vi "number1-state machine.vi"() -> ()   [LabVIEW 2014]
uses:
  number1_global.vi
panel:
  out "Numeric":i32
  out "index of element":i32
  out "Logined":bool
  in  "stop":bool
  out "array":bool[](array[boolean])
  in  "Button":T1
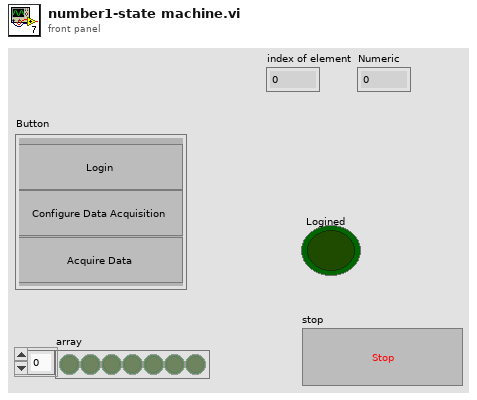
[diagram p1: front panel]
types:
  T1 = cluster{"OK Button":bool, "OK Button 2":bool, "OK Button 3":bool}
  T2 = enum32{"Invalid", "Standard", "Closed", "Hidden", "Minimized", "Maximized"}
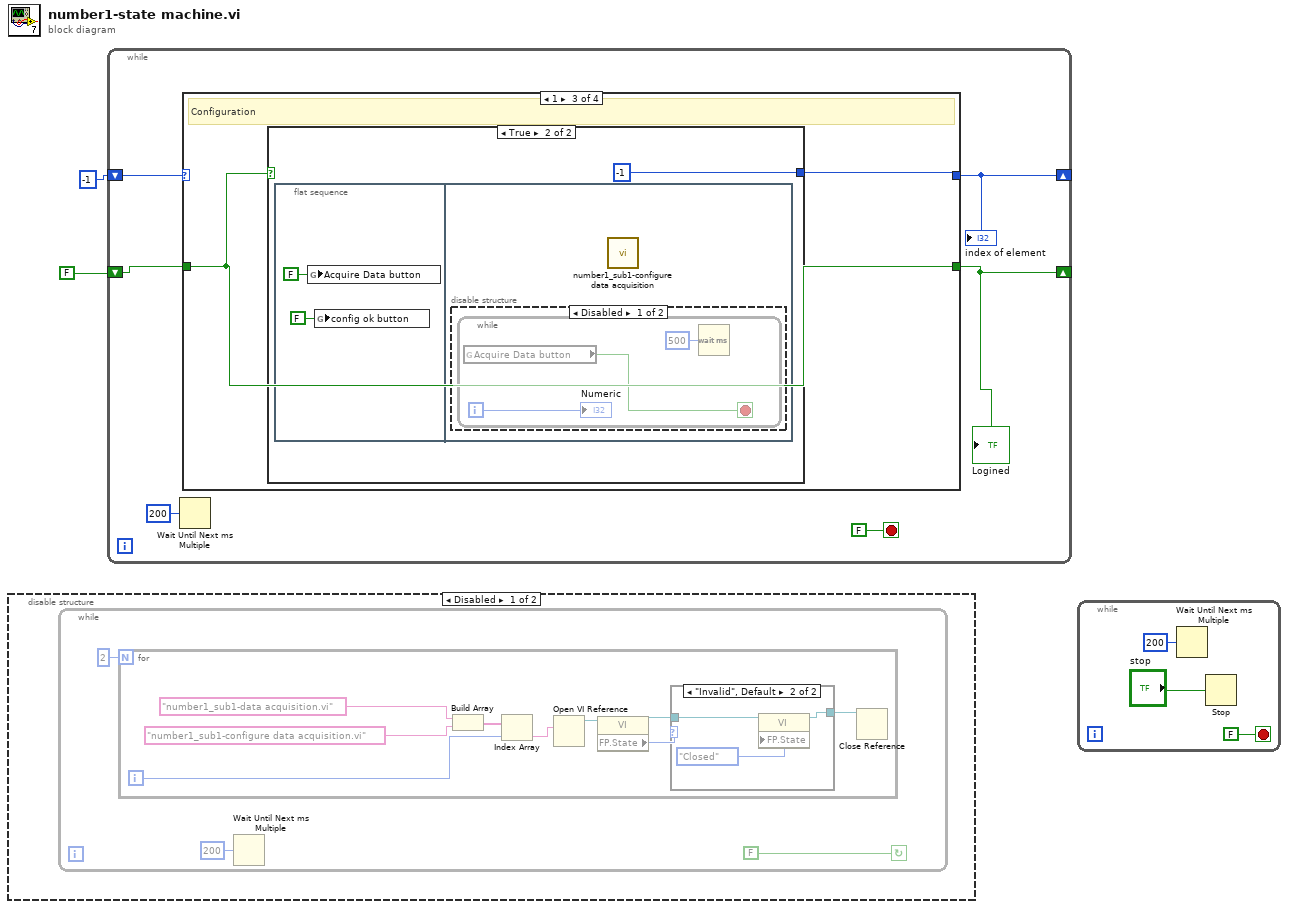
[diagram p0: block diagram]
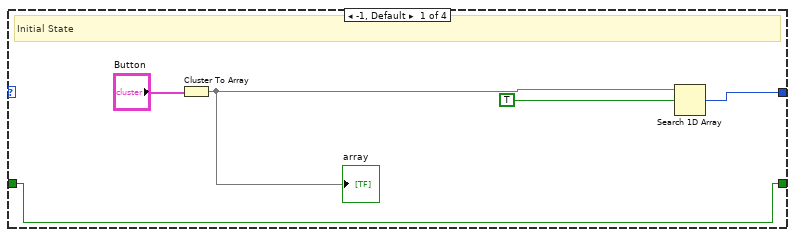
[diagram p4: hidden frame]
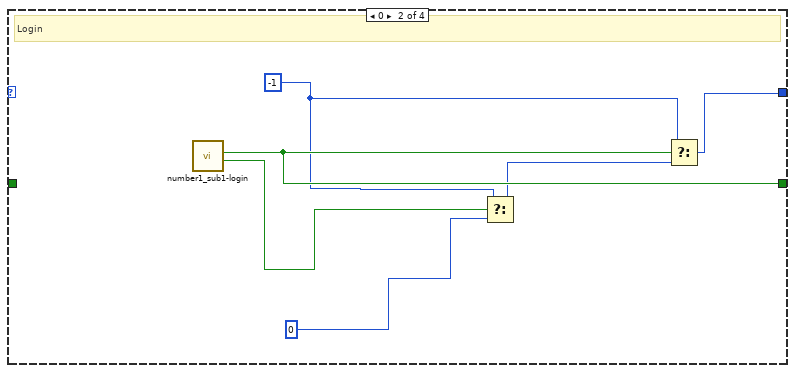
[diagram p5: hidden frame]
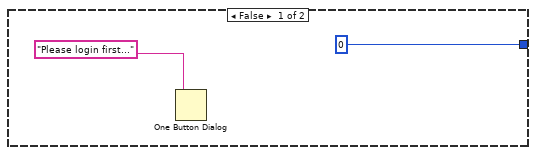
[diagram p6: hidden frame]
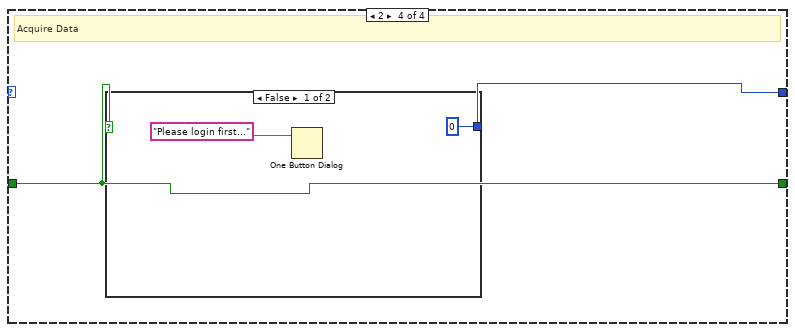
[diagram p8: hidden frame]
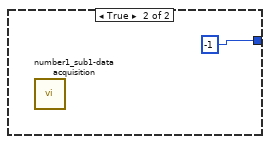
[diagram p9: hidden frame]
diagram:
  n1 = disable-structure shown="Disabled" {
    frame Disabled {
      n2 = while {
        stop <- FALSE continue-if-true
        n3 = for {
          N: 2 -> [_]
          i -> [w12]
          n4 = Build Array("number1_sub1-data acquisition.vi", "number1_sub1-configure data acquisition.vi") -> (w11:string[])
          n5 = Index Array(array=w11, index=w12) -> (element=w10:string)
          n6 = Open VI Reference(vi path=w10) -> (vi reference=w9:refnum<vi>)  [unwired: 5 in, 1 out]
          n7 = property class="VI"(reference=w9) -> (reference out=w7:refnum<vi>, "FP.State"=w8:T2)  [unwired: 1 in, 1 out]
          n8 = case shown="\"Invalid\", Default" w8 {
            tunnel: w7 -> [w15 w17]
            tunnel: [w15 w16] -> w6
            frame "Closed" {
            }
            frame "Invalid", Default {
              n9 = property class="VI"(reference=w17, "FP.State"=T2."Closed" ("Front Panel Window:State")) -> (reference out=w16:refnum<vi>)  [unwired: 1 in, 1 out]
            }
          }
          n10 = Close Reference(reference=w6) -> ()  [unwired: 1 in, 1 out]
        }
        n11 = Wait Until Next ms Multiple(millisecond multiple=u32 200) -> ()  [unwired: 1 out]
      }
    }
    frame Enabled {
    }
  }
  n12 = while {
    shift-right: [w23] -> _
    shift-left: -1 -> [w24]
    shift-right: [w22] -> _
    shift-left: FALSE -> [w21]
    stop <- FALSE stop-if-true
    n13 = Wait Until Next ms Multiple(millisecond multiple=u32 200) -> ()  [unwired: 1 out]
    n14 = case shown="1" w24 {
      tunnel: [w26 w34 w36 w46] -> w23
      tunnel: [w25 w35 w37 w47] -> w22
      tunnel: w21 -> [w25 _ w37 w47]
      frame -1, Default {
        # "Initial State"
        n15 = Cluster To Array(cluster="Button") -> (array=w28:bool[])
        "array" <- w28
        n16 = Search 1D Array(1D array=w28, element=TRUE) -> (index of element=w26:i32)  [unwired: 1 in]
      }
      frame 0 {
        w32 = -1
        # "Login"
        n17 = call "number1_sub1-login.vi"() -> ("UserCancelled"=w33:bool, "Correct"=w35:bool)  [unwired: 10 in]
        n18 = Select(t=w32, s=w33, f=0) -> (s? t:f=w30:i32)
        n19 = Select(t=w32, s=w35, f=w30) -> (s? t:f=w34:i32)
      }
      frame 1 {
        # "Configuration"
        n20 = case shown="True" w37 {
          tunnel: [0 -1] -> w36
          frame False {
            n21 = One Button Dialog(message="Please login first...") -> ()  [unwired: 1 in, 1 out]
          }
          frame True {
            n22 = flat-sequence {
              frame #0 {
                n23 = global write "number1_global.vi" "Acquire Data button"(FALSE ("Acquire Data button")) -> ()
                n24 = global write "number1_global.vi" "config ok button"(FALSE ("config ok button")) -> ()
              }
              frame #1 {
                n25 = disable-structure shown="Disabled" {
                  frame Disabled {
                    n26 = while {
                      i -> [w45]
                      stop <- w43 stop-if-true
                      n27 = global read "number1_global.vi" "Acquire Data button"() -> (w43:bool)
                      n28 = Wait (ms)(milliseconds to wait=u32 500) -> ()  [unwired: 1 out]
                      "Numeric" <- w45
                    }
                  }
                  frame Enabled {
                  }
                }
                n29 = call "number1_sub1-configure data acquisition.vi"() -> ()  [unwired: 8 in]
              }
            }
          }
        }
      }
      frame 2 {
        # "Acquire Data"
        n30 = case shown="False" w47 {
          tunnel: [0 -1 ("index of element")] -> w46
          frame False {
            n31 = One Button Dialog(message="Please login first...") -> ()  [unwired: 1 in, 1 out]
          }
          frame True {
            n32 = call "number1_sub1-data acquisition.vi"() -> ()  [unwired: 5 in, 1 out]
          }
        }
      }
    }
    "Logined" <- w22
    "index of element" <- w23
  }
  n33 = while {
    stop <- FALSE stop-if-true
    n34 = Wait Until Next ms Multiple(millisecond multiple=u32 200) -> ()  [unwired: 1 out]
    n35 = Stop(stop? (T)="stop") -> ()
  }
